vi "Startup.vi"(7 "App":refnum<class>, 8 "error in (no error)":errorcluster, 10 "Config":refnum<class>, 11 "Database in":refnum<class "Database.lvclass">) -> (0 "error out":errorcluster, 3 "Database out":refnum<class "Database.lvclass">)   [LabVIEW 2022 SP3, in "Database.lvclass"]
doc: "Developed by Kevin Thompson\nkevin@thompsonengineering.net\n\nCopyright 2018\nThompson Engineering, LLC"
uses:
  Database.lvclass
  DataTypes/Dependency--cluster.ctl
  Database.lvclass/Database.ctl
  Accessors/Set Dependency.vi
  Accessors/Set VISA Ref.vi
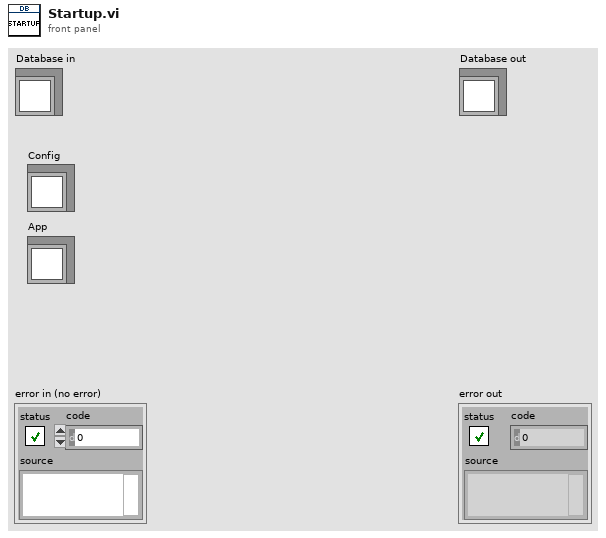
[diagram p1: front panel]
types:
  T1 = typedef "Database.lvclass/Dependency--cluster.ctl" = cluster{"Config":refnum<class>, "ClassRef":refnum<class>}
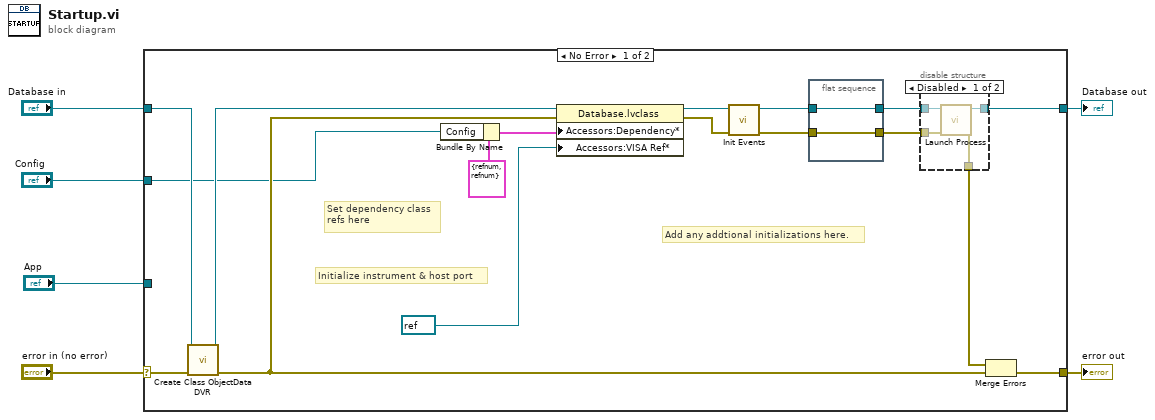
[diagram p0: block diagram]
diagram:
  n1 = case shown="No Error" "error in (no error)" {
    selector: "error in (no error)" -> [w23 w33]
    tunnel: [w16 w33] -> w5
    tunnel: [w13 w32] -> w3
    tunnel: "Database in" -> [w21 w32]
    tunnel: "Config" -> [w8 _]
    tunnel: "App" -> [_ _]
    frame No Error {
      # "Set dependency class\nrefs here"
      # "Initialize instrument & host port"
      # "Add any addtional initializations here."
      n2 = call "Create Class ObjectData DVR.vi"("error in (no error)"=w23, "Database in"=w21) -> ("error out"=w11:errorcluster, "Database out"=w20:refnum<class "Database.lvclass">)  [unwired: 8 in]
      n3 = Bundle By Name(cluster=T1 {"Config"=refnum, "ClassRef"=refnum} ("Dependency"), "Config"=w8) -> (w7:T1)
      n4 = property class="Database.lvclass"(reference=w20, error in=w11, "Accessors:Dependency*"=w7, "Accessors:VISA Ref*"=refnum<visa-resource-name> refnum ("VISA Ref*")) -> (reference out=w22:refnum<class "Database.lvclass">, error out=w19:errorcluster)
      n5 = call "Init Events.vi"("error in (no error)"=w19, "Database in"=w22) -> ("error out"=w17:errorcluster, "Database out"=w18:refnum<class "Database.lvclass">)  [unwired: 8 in]
      n6 = flat-sequence {
        tunnel: w18 -> [w31]
        tunnel: [w31] -> w14
        tunnel: w17 -> [w30]
        tunnel: [w30] -> w15
        frame #0 {
        }
      }
      n7 = disable-structure shown="Disabled" {
        disable-tunnel: w15 -> [w27 w28]
        disable-tunnel: w14 -> [w26 w29]
        disable-tunnel: [w25 w29] -> w13
        disable-tunnel: [w24 w28] -> w12
        frame Disabled {
          n8 = call "Launch Process.vi"("error in (no error)"=w27, "Database in"=w26) -> ("error out"=w24:errorcluster, "Database out"=w25:refnum<class "Database.lvclass">)  [unwired: 6 in, 2 out]
        }
        frame Enabled {
        }
      }
      n9 = Merge Errors(w12, w11) -> (w16:errorcluster)
    }
    frame Error {
    }
  }
  "error out" <- w5
  "Database out" <- w3
